vi "TangensFilter3.vi"(4 "error IN":errorcluster, 6 "Max Angle":dbl, 7 "[IN] Finded Chains (X,Y,dX,dY)":dbl[][](array[numeric])) -> (0 "error OUT":errorcluster, 1 "[OUT] Filtered Chains (X,Y,dX,dY)":dbl[][](array[numeric]))   [LabVIEW 2013]
doc: "Implementation of following simple filter: if further displacement has the angle more than maximal, then such displacement will be deleted"
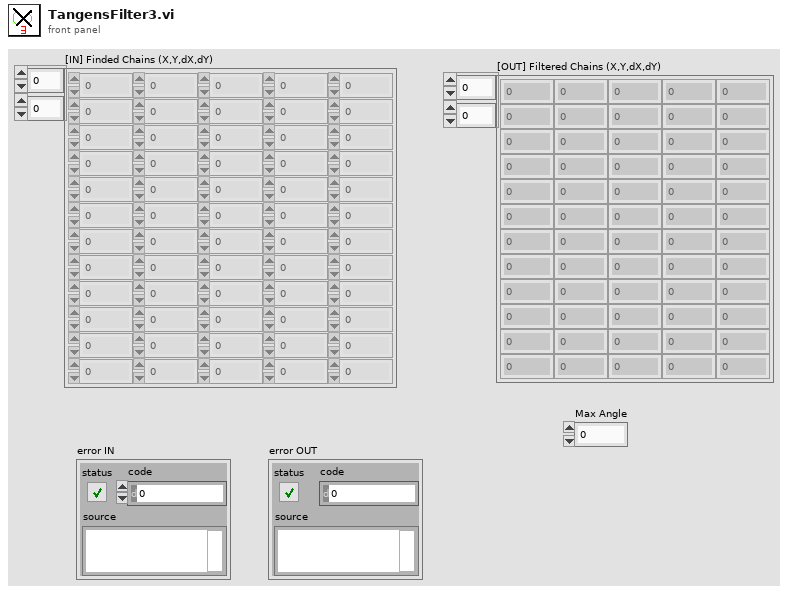
[diagram p1: front panel]
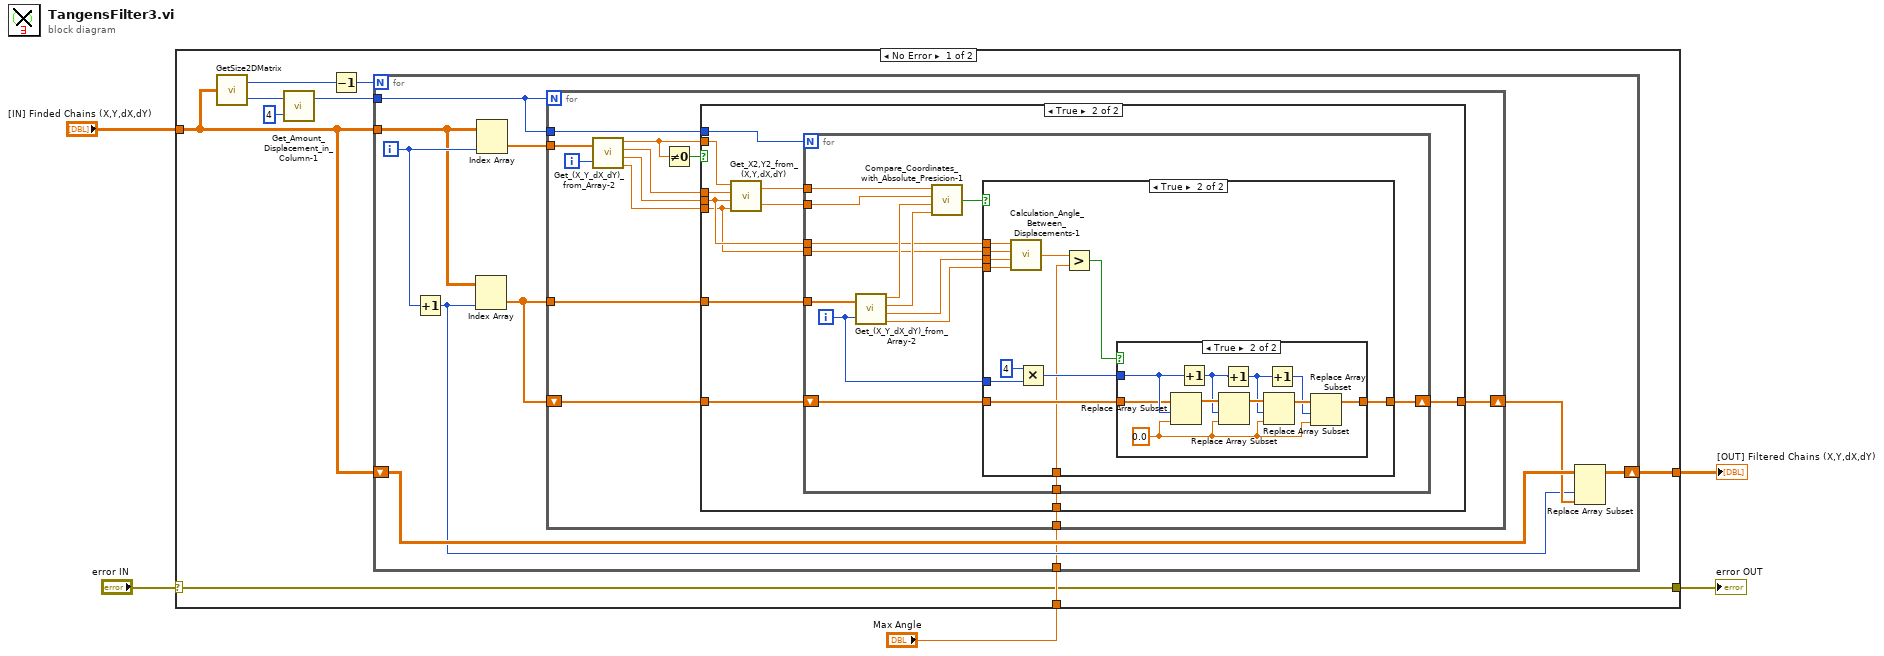
[diagram p0: block diagram]
diagram:
  n1 = case shown="No Error" "error IN" {
    selector: "error IN" -> [w6 w88]
    tunnel: [w13 w87] -> w5
    tunnel: "[IN] Finded Chains (X,Y,dX,dY)" -> [w12 w87]
    tunnel: "Max Angle" -> [w7 _]
    tunnel: [w6 w88] -> w1
    frame No Error {
      n2 = call "GetSize2DMatrix.vi"("Array IN (2D)"=w12) -> ("# Cols"=w11:i32, "# Rows"=w9:i32)
      n3 = call "Get_Amount_Displacement_in_Column-1.vi"("multiplier"=4, "# Rows"=w9) -> ("Displ amount"=w8:i32)  [unwired: 1 out]
      n4 = Decrement(x=w11) -> (x-1=w14:i32)
      n5 = for {
        N: w14 -> [_]
        tunnel: w12 -> [w22]
        shift-right: [w17] -> w13
        shift-left: w12 -> [w20]
        tunnel: w8 -> [w16]
        tunnel: w7 -> [w15]
        i -> [w23]
        n6 = Increment(x=w23) -> (x+1=w18:i32)
        n7 = Index Array(array=w22, index (col)=w18) -> (element=w21:dbl[])  [unwired: 1 in]
        n8 = Index Array(array=w22, index (col)=w23) -> (element=w24:dbl[])  [unwired: 1 in]
        n9 = for {
          N: w16 -> [_]
          tunnel: w24 -> [w31]
          tunnel: w16 -> [w35]
          tunnel: w21 -> [w34]
          shift-right: [w32] -> w19
          shift-left: w21 -> [w33]
          tunnel: w15 -> [w25]
          i -> [w30]
          n10 = call "Get_(X_Y_dX_dY)_from_Array-2.vi"("(X,Y,dX,dY)"=w31, "Index of Displacement"=w30) -> ("X"=w29:dbl, "Y"=w28:dbl, "dX"=w27:dbl, "dY"=w26:dbl)
          n11 = Not Equal To 0?(x=w29) -> (x != 0?=w36:bool)
          n12 = case shown="True" w36 {
            tunnel: w35 -> [_ w48]
            tunnel: w29 -> [_ w44]
            tunnel: w34 -> [_ w47]
            tunnel: w33 -> [w37 w46]
            tunnel: [w37 w45] -> w32
            tunnel: w28 -> [_ w43]
            tunnel: w27 -> [_ w40]
            tunnel: w26 -> [_ w39]
            tunnel: w25 -> [_ w38]
            frame False {
            }
            frame True {
              n13 = call "Get_X2,Y2_from_(X,Y,dX,dY).vi"("dY"=w39, "dX"=w40, "Y1"=w43, "X1"=w44) -> ("Y2 = (Y1+dY)"=w41:dbl, "X2 = (X1+dX)"=w42:dbl)
              n14 = for {
                N: w48 -> [_]
                tunnel: w47 -> [w60]
                shift-right: [w61] -> w45
                shift-left: w46 -> [w62]
                tunnel: w42 -> [w59]
                tunnel: w41 -> [w58]
                tunnel: w40 -> [w54]
                tunnel: w39 -> [w53]
                tunnel: w38 -> [w49]
                i -> [w50]
                n15 = call "Get_(X_Y_dX_dY)_from_Array-2.vi"("(X,Y,dX,dY)"=w60, "Index of Displacement"=w50) -> ("X"=w57:dbl, "Y"=w56:dbl, "dX"=w52:dbl, "dY"=w51:dbl)
                n16 = call "Compare_Coordinates_with_Absolute_Presicion-1.vi"("X 1"=w59, "Y 1"=w58, "X 2"=w57, "Y 2"=w56) -> ("[OUT] Same coordinates?"=w55:bool)  [unwired: 1 in]
                n17 = case shown="True" w55 {
                  tunnel: w62 -> [w63 w67]
                  tunnel: [w63 w66] -> w61
                  tunnel: w54 -> [_ w75]
                  tunnel: w53 -> [_ w74]
                  tunnel: w52 -> [_ w73]
                  tunnel: w51 -> [_ w72]
                  tunnel: w50 -> [_ w70]
                  tunnel: w49 -> [_ w65]
                  frame False {
                  }
                  frame True {
                    n18 = call "Calculation_Angle_Between_Displacements-1.vi"("dY 2"=w72, "dX 2"=w73, "dY 1"=w74, "dX 1"=w75) -> ("angle in degrees"=w71:dbl)
                    n19 = Multiply(x=4, y=w70) -> (x*y=w68:i32)
                    n20 = Greater?(x=w71, y=w65) -> (0:w64:bool)
                    n21 = case shown="True" w64 {
                      tunnel: w68 -> [_ w79]
                      tunnel: w67 -> [w76 w78]
                      tunnel: [w76 w77] -> w66
                      frame False {
                      }
                      frame True {
                        w83 = 0.0 ("new element/subarray")
                        n22 = Replace Array Subset(array=w78, new element=w83, index=w79) -> (w86:dbl[])
                        n23 = Increment(x=w79) -> (x+1=w82:i32)
                        n24 = Replace Array Subset(array=w86, new element=w83, index=w82) -> (w85:dbl[])
                        n25 = Increment(x=w82) -> (x+1=w81:i32)
                        n26 = Replace Array Subset(array=w85, new element=w83, index=w81) -> (w84:dbl[])
                        n27 = Increment(x=w81) -> (x+1=w80:i32)
                        n28 = Replace Array Subset(array=w84, new element=w83, index=w80) -> (w77:dbl[])
                      }
                    }
                  }
                }
              }
            }
          }
        }
        n29 = Replace Array Subset(array=w20, new element=w19, index (col)=w18) -> (w17:dbl[][])  [unwired: 1 in]
      }
    }
    frame Error {
    }
  }
  "[OUT] Filtered Chains (X,Y,dX,dY)" <- w5
  "error OUT" <- w1
